vi "Fetch (Scaled).vi"(0 "VISA resource name":refnum<visa-resource-name>, 1 "Segment Index (0)":i32 format="%.0g", 5 "Measurement Source (1: Channel 1)":i32(ring)=1 items=["Channel 1"=1, "Channel 2"=2, "Channel 3"=3, "Channel 4"=4, "Function 1"=5, "Function 2"=6, "Function 3"=7, "Function 4"=8, "Memory 1"=9, "Memory 2"=10, "Memory 3"=11, "Memory 4"=12], 7 "Number of Samples (1000)":i32=10000 caption="Number of Samples (10000)", 9 "Maximum Time (10000ms)":u32=10000, 11 "error in (no error)":errorcluster, 12 "Offset (0)":i32) -> (4 "VISA resource name out":refnum<visa-resource-name>, 6 "Waveform Information":T1, 8 "Waveform Data":dbl[](array[numeric]), 15 "error out":errorcluster)   [LabVIEW 2020, in "Agilent 90000 Series.lvlib"]
doc: "Fetches the scaled waveform from instrument. Use this VI under either word data format or byte data format configuration."
uses:
  Agilent 90000 Series.lvlib
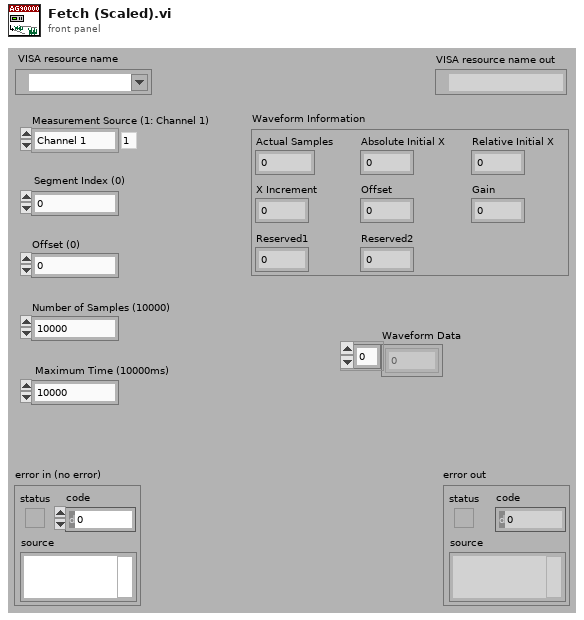
[diagram p1: front panel]
types:
  T1 = cluster{"Actual Samples":i32, "Absolute Initial X":dbl, "Relative Initial X":dbl, "X Increment":dbl, "Offset":dbl, "Gain":dbl, "Reserved1":dbl, "Reserved2":dbl}
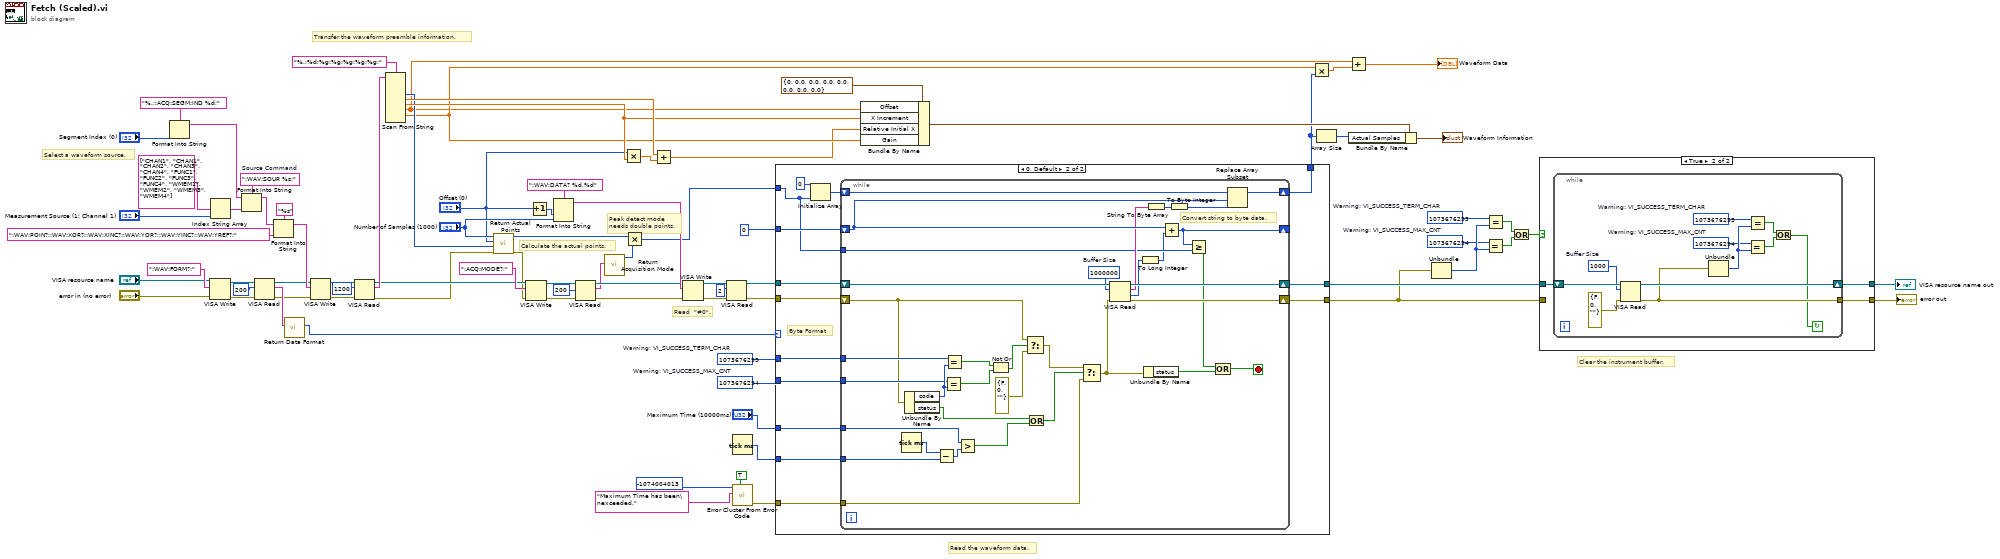
[diagram p0: block diagram]
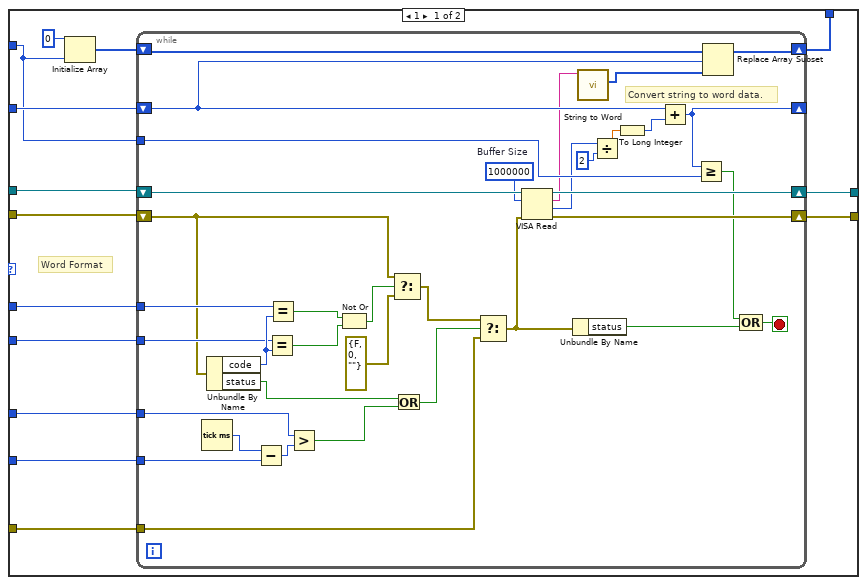
[diagram p2: hidden frame]
diagram:
  w47 = 1073676294  # Warning: VI_SUCCESS_MAX_CNT
  w48 = 1073676293  # Warning: VI_SUCCESS_TERM_CHAR
  w66 = 1073676294  # Warning: VI_SUCCESS_MAX_CNT
  w65 = 1073676293  # Warning: VI_SUCCESS_TERM_CHAR
  w79 = ":WAV:SOUR %s;"  # Source Command
  # "Peak detect mode\nneeds double points."
  # "Calculate the actual points."
  # "Read  \"#0\"."
  # "Transfer the waveform preamble information."
  # "Select a waveform source."
  # "Clear the instrument buffer."
  # "Read the waveform data."
  n1 = Format Into String(format string="%.;:ACQ:SEGM:IND %d;", "Segment Index (0)") -> (resulting string=w1:string)  [unwired: 2 in, 1 out]
  n2 = VISA Write(VISA resource name="VISA resource name", write buffer=":WAV:FORM?;", error in (no error)="error in (no error)") -> (VISA resource name out=w40:refnum<visa-resource-name>, error out=w39:errorcluster)  [unwired: 1 out]
  n3 = Index String Array(1:"Measurement Source (1: Channel 1)", 2:string[] ["CHAN1", "CHAN1", "CHAN2", "CHAN3", "CHAN4", "FUNC1", "FUNC2", "FUNC3", "FUNC4", "WMEM1", "WMEM2", "WMEM3", "WMEM4"] ("subarray 2")) -> (0:w74:string)  [unwired: 1 out]
  n4 = Format Into String(format string=w79, initial string=w1, w74) -> (resulting string=w77:string)  [unwired: 1 in, 1 out]
  n5 = VISA Read(VISA resource name=w40, byte count=u32 200, error in (no error)=w39) -> (VISA resource name out=w34:refnum<visa-resource-name>, read buffer=w30:string, error out=w6:errorcluster)  [unwired: 1 out]
  n6 = Format Into String(format string="%s", initial string=w77, ":WAV:POIN?;:WAV:XOR?;:WAV:XINC?;:WAV:YOR?;:WAV:YINC?;:WAV:YREF?;") -> (resulting string=w76:string)  [unwired: 1 in, 1 out]
  n7 = call "Return Data Format.vi"("String In"=w30) -> ("Data Format"=w5:u16)  [unwired: 1 in, 9 out]
  n8 = VISA Write(VISA resource name=w34, write buffer=w76, error in (no error)=w6) -> (VISA resource name out=w82:refnum<visa-resource-name>, error out=w81:errorcluster)  [unwired: 1 out]
  n9 = VISA Read(VISA resource name=w82, byte count=u32 1200, error in (no error)=w81) -> (VISA resource name out=w23:refnum<visa-resource-name>, read buffer=w60:string, error out=w12:errorcluster)  [unwired: 1 out]
  n10 = Scan From String(format string="%.;%d;%g;%g;%g;%g;%g;", input string=w60) -> (output 1=w26:i32, output 2=w29:dbl, output 3=w28:dbl, output 4=w8:dbl, output 5=w19:dbl)  [unwired: 2 in, 10 out]
  n11 = call "Return Actual Points.vi"("error in (no error)"=w12, "Total Points (2000)"=w26, "Offset (0)"="Offset (0)", "Number of Samples (1000)"="Number of Samples (1000)") -> ("error out"=w11:errorcluster, "Actual Points"=w24:i32)  [unwired: 6 out]
  n12 = VISA Write(VISA resource name=w23, write buffer=":ACQ:MODE?;", error in (no error)=w11) -> (VISA resource name out=w53:refnum<visa-resource-name>, error out=w54:errorcluster)  [unwired: 1 out]
  n13 = Increment(x="Offset (0)") -> (x+1=w9:i32)
  n14 = Format Into String(format string=":WAV:DATA? %d,%d", w9, "Number of Samples (1000)") -> (resulting string=w57:string)  [unwired: 2 in, 1 out]
  n15 = VISA Read(VISA resource name=w53, byte count=u32 200, error in (no error)=w54) -> (VISA resource name out=w52:refnum<visa-resource-name>, read buffer=w13:string, error out=w51:errorcluster)  [unwired: 1 out]
  n16 = call "Return Acquisition Mode.vi"("Acquisition Mode"=w13) -> ("Multiply Factor"=w14:i32)  [unwired: 10 out]
  n17 = Multiply(x="Offset (0)", y=w28) -> (x*y=w56:dbl)
  n18 = Multiply(x=w24, y=w14) -> (x*y=w25:i32)
  n19 = Add(x=w29, y=w56) -> (x+y=w7:dbl)
  n20 = VISA Write(VISA resource name=w52, write buffer=w57, error in (no error)=w51) -> (VISA resource name out=w63:refnum<visa-resource-name>, error out=w62:errorcluster)  [unwired: 1 out]
  n21 = VISA Read(VISA resource name=w63, byte count=u32 2, error in (no error)=w62) -> (VISA resource name out=w31:refnum<visa-resource-name>, error out=w32:errorcluster)  [unwired: 2 out]
  n22 = Tick Count (ms)() -> (millisecond timer value=w45:u32)
  n23 = call <vilib>:"Error Cluster From Error Code.vi"("show call chain? (False)"=TRUE, "error message (\"\")"="Maximum Time has been\nexceeded." ("error message (\"\")"), "error code (0)"=-1074004013) -> ("error out"=w42:errorcluster)  [unwired: 1 in, 5 out]
  n24 = case shown="0, Default" w5 {
    tunnel: [w96 w146] -> w72
    tunnel: [w95 w145] -> w71
    tunnel: w32 -> [w94 w144]
    tunnel: w31 -> [w93 w143]
    tunnel: [w92 w142] -> w15
    tunnel: w48 -> [w91 w141]
    tunnel: w47 -> [w90 w140]
    tunnel: "Maximum Time (10000ms)" -> [w89 w139]
    tunnel: w45 -> [w88 w138]
    tunnel: w42 -> [w87 w137]
    tunnel: w25 -> [w83 w133]
    tunnel: 0 ("index") -> [w86 w136]
    frame 1 {
      # "Word Format"
      n25 = Initialize Array(i16 0 ("element"), w83) -> (w84:i16[])
      n26 = while {
        shift-right: [w128] -> w95
        shift-left: w94 -> [w116]
        shift-right: [w132] -> w96
        shift-left: w93 -> [w131]
        shift-right: [w129] -> w92
        shift-left: w84 -> [w103]
        shift-right: [w126] -> _
        shift-left: w86 -> [w127]
        tunnel: w83 -> [w125]
        tunnel: w91 -> [w118]
        tunnel: w90 -> [w117]
        tunnel: w89 -> [w113]
        tunnel: w88 -> [w112]
        tunnel: w87 -> [w107]
        stop <- w104 stop-if-true
        w130 = u32 1000000  # Buffer Size
        # "Convert string to word data."
        n27 = Tick Count (ms)() -> (millisecond timer value=w114:u32)
        n28 = Unbundle By Name(w116) -> ("code"=w119:i32, "status"=w111:bool)
        n29 = Subtract(x=w114, y=w112) -> (x-y=w115:u32)
        n30 = Equal?(x=w117, y=w119) -> (x = y?=w122:bool)
        n31 = Equal?(x=w118, y=w119) -> (x = y?=w123:bool)
        n32 = Greater?(x=w113, y=w115) -> (0:w110:bool)
        n33 = Not Or(1:w122, 2:w123) -> (0:w121:bool)
        n34 = Select(t=w116, s=w121, f=errorcluster {"status"=FALSE, "code"=0, "source"=""} ("error in (no error)")) -> (s? t:f=w109:errorcluster)
        n35 = Or(x=w111, y=w110) -> (x .or. y?=w108:bool)
        n36 = Select(t=w109, s=w108, f=w107) -> (s? t:f=w106:errorcluster)
        n37 = VISA Read(VISA resource name=w131, byte count=w130, error in (no error)=w106) -> (VISA resource name out=w132:refnum<visa-resource-name>, read buffer=w97:string, return count=w101:u32, error out=w128:errorcluster)
        n38 = Unbundle By Name(w106) -> ("status"=w105:bool)
        n39 = call "String to Word.vi"("String"=w97) -> ("Int16 Data"=w98:i16[])  [unwired: 1 in, 9 out]
        n40 = Divide(x=w101, y=u32 2) -> (x/y=w102:dbl)
        n41 = To Long Integer(number=w102) -> (32bit integer=w99:i32)
        n42 = Add(x=w127, y=w99) -> (x+y=w126:i32)
        n43 = Greater Or Equal?(x=w126, y=w125) -> (x >= y?=w124:bool)
        n44 = Replace Array Subset(array=w103, new element=w98, index=w127) -> (w129:i16[])
        n45 = Compound Arithmetic op=OR(w124, w105) -> (w104:bool)
      }
    }
    frame 0, Default {
      # "Byte Format"
      n46 = Initialize Array(i8 0 ("element"), w133) -> (w134:i8[])
      n47 = while {
        shift-right: [w177] -> w145
        shift-left: w144 -> [w165]
        shift-right: [w181] -> w146
        shift-left: w143 -> [w180]
        shift-right: [w178] -> w142
        shift-left: w134 -> [w152]
        shift-right: [w174] -> _
        shift-left: w136 -> [w175]
        tunnel: w141 -> [w167]
        tunnel: w140 -> [w166]
        tunnel: w139 -> [w162]
        tunnel: w138 -> [w161]
        tunnel: w137 -> [w156]
        tunnel: w133 -> [w149]
        stop <- w153 stop-if-true
        w179 = u32 1000000  # Buffer Size
        # "Convert string to byte data."
        n48 = Tick Count (ms)() -> (millisecond timer value=w163:u32)
        n49 = Unbundle By Name(w165) -> ("code"=w168:i32, "status"=w160:bool)
        n50 = Subtract(x=w163, y=w161) -> (x-y=w164:u32)
        n51 = Equal?(x=w166, y=w168) -> (x = y?=w171:bool)
        n52 = Equal?(x=w167, y=w168) -> (x = y?=w172:bool)
        n53 = Greater?(x=w162, y=w164) -> (0:w159:bool)
        n54 = Not Or(1:w171, 2:w172) -> (0:w170:bool)
        n55 = Select(t=w165, s=w170, f=errorcluster {"status"=FALSE, "code"=0, "source"=""} ("error in (no error)")) -> (s? t:f=w158:errorcluster)
        n56 = Or(x=w160, y=w159) -> (x .or. y?=w157:bool)
        n57 = Select(t=w158, s=w157, f=w156) -> (s? t:f=w155:errorcluster)
        n58 = VISA Read(VISA resource name=w180, byte count=w179, error in (no error)=w155) -> (VISA resource name out=w181:refnum<visa-resource-name>, read buffer=w151:string, return count=w176:u32, error out=w177:errorcluster)
        n59 = To Long Integer(number=w176) -> (32bit integer=w147:i32)
        n60 = Unbundle By Name(w155) -> ("status"=w154:bool)
        n61 = String To Byte Array(string=w151) -> (unsigned byte array=w150:u8[])
        n62 = Add(x=w175, y=w147) -> (x+y=w174:i32)
        n63 = To Byte Integer(number=w150) -> (8bit integer=w148:i8[])
        n64 = Greater Or Equal?(x=w174, y=w149) -> (x >= y?=w173:bool)
        n65 = Compound Arithmetic op=OR(w173, w154) -> (w153:bool)
        n66 = Replace Array Subset(array=w152, new element=w148, index=w175) -> (w178:i8[])
      }
    }
  }
  n67 = Bundle By Name(cluster=T1 {"Actual Samples"=0, "Absolute Initial X"=0.0, "Relative Initial X"=0.0, "X Increment"=0.0, "Offset"=0.0, "Gain"=0.0, "Reserved1"=0.0, "Reserved2"=0.0} ("Waveform Information"), "Offset"=w8, "X Increment"=w28, "Relative Initial X"=w7, "Gain"=w19) -> (w55:T1)
  n68 = Multiply(x=w19, y=w15) -> (x*y=w50:dbl[])
  n69 = Array Size(array=w15) -> (size(s)=w16:i32)
  n70 = Add(x=w8, y=w50) -> (x+y=→"Waveform Data":dbl[])
  n71 = Bundle By Name(cluster=w55, "Actual Samples"=w16) -> (→"Waveform Information":T1)
  n72 = Unbundle(w71) -> ("code"=w67:i32)  [unwired: 2 out]
  n73 = Equal?(x=w66, y=w67) -> (x = y?=w69:bool)
  n74 = Equal?(x=w65, y=w67) -> (x = y?=w70:bool)
  n75 = Or(x=w70, y=w69) -> (x .or. y?=w68:bool)
  n76 = case shown="True" w68 {
    tunnel: w72 -> [w183 w186]
    tunnel: w71 -> [w182 _]
    tunnel: [w183 w185] -> w21
    tunnel: [w182 w184] -> w20
    frame False {
    }
    frame True {
      n77 = while {
        shift-right: [w196] -> w185
        shift-left: w186 -> [w197]
        tunnel: [w189] -> w184
        stop <- w188 continue-if-true
        w191 = 1073676294  # Warning: VI_SUCCESS_MAX_CNT
        w190 = 1073676293  # Warning: VI_SUCCESS_TERM_CHAR
        w195 = u32 1000  # Buffer Size
        n78 = VISA Read(VISA resource name=w197, byte count=w195, error in (no error)=errorcluster {"status"=FALSE, "code"=0, "source"=""}) -> (VISA resource name out=w196:refnum<visa-resource-name>, error out=w189:errorcluster)  [unwired: 2 out]
        n79 = Unbundle(w189) -> ("code"=w192:i32)  [unwired: 2 out]
        n80 = Equal?(x=w191, y=w192) -> (x = y?=w193:bool)
        n81 = Equal?(x=w190, y=w192) -> (x = y?=w194:bool)
        n82 = Or(x=w194, y=w193) -> (x .or. y?=w188:bool)
      }
    }
  }
  "error out" <- w20
  "VISA resource name out" <- w21
